vi "Initialize.vi"(8 "error in (no error)":errorcluster, 10 "DMM Alias":string) -> (0 "error out":errorcluster, 3 "DMM out":refnum<class "DMM.lvclass">)   [LabVIEW 2020, in "DMM.lvclass"]
uses:
  DMM.lvclass
  DMM.lvclass/DMM.ctl
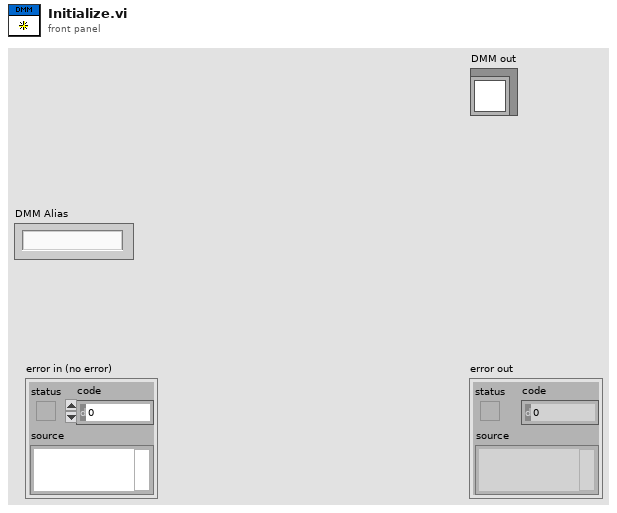
[diagram p1: front panel]
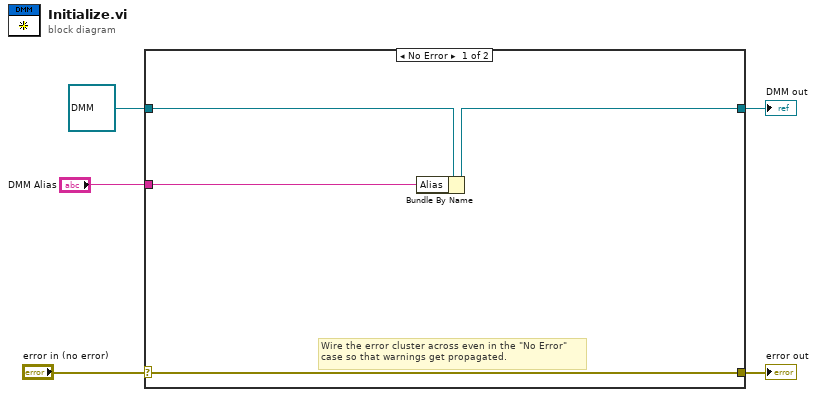
[diagram p0: block diagram]
diagram:
  n1 = case shown="No Error" "error in (no error)" {
    selector: "error in (no error)" -> [w8 w11]
    tunnel: [w8 w11] -> w4
    tunnel: [w7 w10] -> w2
    tunnel: refnum<class "DMM.lvclass"> refnum ("DMM in") -> [w9 w10]
    tunnel: "DMM Alias" -> [w6 _]
    frame No Error {
      # "Wire the error cluster across even in the \"No Error\"\ncase so that warnings get propagated."
      n2 = Bundle By Name(cluster=w9, "Alias"=w6) -> (w7:refnum<class "DMM.lvclass">)
    }
    frame Error {
    }
  }
  "error out" <- w4
  "DMM out" <- w2
